vi "load_arbitrary_waveform.vi"() -> ()   [LabVIEW 2016]
uses:
  <vilib>/Utility/file.llb/Read Delimited Spreadsheet (DBL).vi
  <instrlib>/Agilent 33XXX Series/Agilent 33XXX Series.lvlib
panel:
  in  "Serial Configuration":T1={"Baud Rate"=9600, "Parity"=0, "Data Bits"=8, "Flow Control"=4} {"Flow Control" items=["None", "XON/XOFF", "RTS/CTS", "XON/XOFF & RTS/CTS", "DTR/DSR", "XON/XOFF & DTR/DSR"]; "Data Bits" items=["7"=7, "8"=8]; "Parity" items=["None", "Odd", "Even", "Mark", "Space"]; "Baud Rate" items=["300"=300, "600"=600, "1200"=1200, "2400"=2400, "4800"=4800, "9600"=9600, "19200"=19200]}
  in  "VISA resource name 2":refnum<visa-resource-name>
  in  "Frequency (1000 Hz)":dbl=1000.0
  in  "Gain (1.0)":dbl=1.0
  in  "Offset (0 V)":dbl
  in  "Arbitrary Waveform Name":string="ARB1"
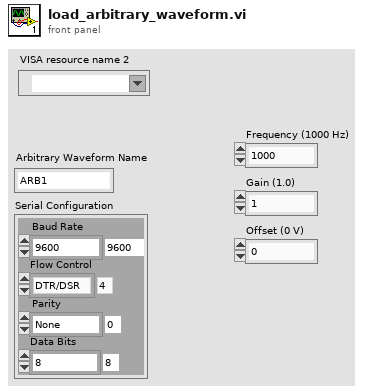
[diagram p1: front panel]
types:
  T1 = cluster{"Baud Rate":u32, "Parity":u16, "Data Bits":u16, "Flow Control":u16}
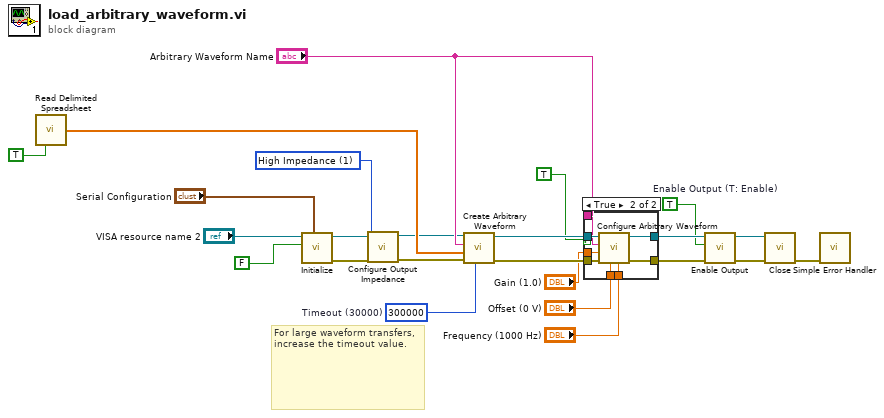
[diagram p0: block diagram]
diagram:
  w2 = u16 1 items=["50 Ohms", "High Impedance", "User Defined"] ("Impedance (0: 50 Ohms)")
  w13 = u32 300000  # Timeout (30000)
  w17 = TRUE  # Enable Output (T: Enable)
  # "For large waveform transfers, increase the timeout value."
  n1 = call-poly <vilib>:"Read Delimited Spreadsheet.vi"("transpose? (F)"=TRUE) -> ("first row"=w7:dbl[])  [unwired: 9 in, 5 out]
  n2 = call <instrlib>:"Initialize.vi"("Serial Configuration"="Serial Configuration", "ID Query (True)"=FALSE, "VISA resource name"="VISA resource name 2") -> ("error out"=w6:errorcluster, "VISA resource name out"=w4:refnum<visa-resource-name>)  [unwired: 7 in]
  n3 = call <instrlib>:"Configure Output Impedance.vi"("error in (no error)"=w6, "Impedance (0: 50 Ohms)"=w2, "VISA resource name"=w4) -> ("error out"=w5:errorcluster, "VISA resource name out"=w3:refnum<visa-resource-name>)  [unwired: 7 in]
  n4 = call <instrlib>:"Create Arbitrary Waveform.vi"("Timeout (10000)"=w13, "error in (no error)"=w5, "Arbitrary Waveform Data"=w7, "Arbitrary Waveform Name (\"ARB1\")"="Arbitrary Waveform Name", "VISA resource name"=w3) -> ("error out"=w22:errorcluster, "VISA resource name out"=w23:refnum<visa-resource-name>)  [unwired: 5 in]
  n5 = case shown="True" TRUE {
    tunnel: w23 -> [w25 w34]
    tunnel: w22 -> [w26 w33]
    tunnel: [w25 w32] -> w21
    tunnel: [w26 w31] -> w20
    tunnel: "Arbitrary Waveform Name" -> [_ w30]
    tunnel: "Gain (1.0)" -> [_ w29]
    tunnel: "Offset (0 V)" -> [_ w28]
    tunnel: "Frequency (1000 Hz)" -> [_ w27]
    frame False {
    }
    frame True {
      n6 = call <instrlib>:"Configure Arbitrary Waveform.vi"("Frequency (1000 Hz)"=w27, "Offset (0.00 V)"=w28, "error in (no error)"=w33, "Gain (1.0)"=w29, "Arbitrary Waveform Name (\"ARB1\")"=w30, "VISA resource name"=w34) -> ("error out"=w31:errorcluster, "VISA resource name out"=w32:refnum<visa-resource-name>)  [unwired: 4 in]
    }
  }
  n7 = call <instrlib>:"Enable Output.vi"("error in (no error)"=w20, "Enable Output  (T: Enable)"=w17, "VISA resource name"=w21) -> ("error out"=w19:errorcluster, "VISA resource name out"=w18:refnum<visa-resource-name>)  [unwired: 7 in]
  n8 = call <instrlib>:"Close.vi"("error in (no error)"=w19, "VISA resource name"=w18) -> ("error out"=w24:errorcluster)  [unwired: 9 in]
  n9 = call <vilib>:"Simple Error Handler.vi"("error in (no error)"=w24) -> ()  [unwired: 4 in, 5 out]
